vi "PH_ImageOperator.Show Beam Analysis.vi"(0 "i ref in":refnum<vi>, 2 "GUI Image In":T1, 5 "error in (no error)":errorcluster) -> (14 "i ref out":refnum<vi>, 16 "GUI Image Out":T1, 19 "error out":errorcluster)   [LabVIEW 2014, in "PH_ImageOperator.lvlib"]
doc: "This VI overlays beam analysis information to the GUI image."
uses:
  PH_ImageOperator.lvlib
  <vilib>/vision/Image Controls.llb/IMAQ Image.ctl
  PH_Image_Common/PH_Image_Common.lvlib
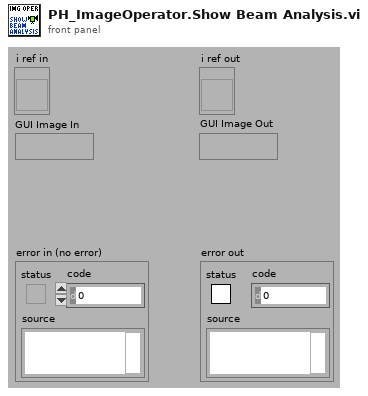
[diagram p1: front panel]
types:
  T1 = typedef "IMAQ Image.ctl" = refnum<image>
  T2 = typedef "PH_ImageOperator.lvlib/PH_ImageOperator.i attribute.ctl" = cluster{"GUI Refs":cluster{"Delete":refnum<vi>, "Calibration status":refnum<vi>, "BI subtracted":refnum<vi>, "calc Energy":refnum<vi>, "Energy: expected value":refnum<vi>, "Energy: Tolerance":refnum<vi>, "Energy calculated":refnum<vi>, "Energy":refnum<vi>, "calc Beam Anal":refnum<vi>, "Maj Diam 1/esquare":refnum<vi>, "Min Diam 1/esquare":refnum<vi>, "Azi Angle":refnum<vi>, "Min/Maj Diam esquare":refnum<vi>, "Beam analysed":refnum<vi>, "CoG - x":refnum<vi>, "CoG - y":refnum<vi>, "BA: Method":refnum<vi>, "BA: Steps":refnum<vi>, "BA: Factor":refnum<vi>, "calc Traces":refnum<vi>, "Traces: Fit Gauss":refnum<vi>, "Traces calculated":refnum<vi>, "Maj FWHM":refnum<vi>, "Min FWHM":refnum<vi>, "Major Trace":refnum<vi>, "Minor Trace":refnum<vi>, "Maj Fit Order":refnum<vi>, "Min Fit Order":refnum<vi>, "Position calculated":refnum<vi>, "Position":refnum<vi>, "Type":refnum<vi>, "Center":refnum<vi>, "exp - X":refnum<vi>, "exp - Y":refnum<vi>, "Tolerance":refnum<vi>, "f":refnum<vi>, "M":refnum<vi>, "D":refnum<vi>, "q":refnum<vi>, "Dummy Method":refnum<vi>, "Dummy Type":refnum<vi>, "Global On":refnum<vi>, "Traces: No offset":refnum<vi>, "Maj 99%":refnum<vi>, "Min 99%":refnum<vi>, "GUI FF Image":refnum<vi>, "calc Fill Factor":refnum<vi>, "FF calculated":refnum<vi>, "Fill Factor: Filter?":refnum<vi>, "FF: Damage Threshold":refnum<vi>, "FF: Threshold":refnum<vi>, "FF: max allow. Energy":refnum<vi>, "FF: Fillfactor":refnum<vi>, "Calibration data":refnum<vi>}, "List of GUIs":string[], "Calibration":cluster{"Status":T3, "Calibration data":T4, "Calibration Data File":path}, "Final Image":cluster{"BI Subtraction Failure":bool}, "Energy":cluster{"on":bool, "expected value [mJ]":dbl, "Tolerance [%]":dbl, "State":T3, "Energy [mJ]":dbl, "Unit":string, "calculated @":timestamp}, "Beam Analysis":cluster{"on":bool, "Data":T5, "Method":bool, "Steps":i32, "Factor":i32, "ROI":cluster{"Left":i32, "Top":i32, "Right":i32, "Bottom":i32}, "analysed @":timestamp}, "Trace Analysis":cluster{"on":bool, "Fit on":bool, "Maj FWHM":dbl, "Min FWHM":dbl, "Maj Fit Order":i32, "Min Fit Order":i32, "No Offset":bool, "Maj 99%":dbl, "Min 99%":dbl, "Traces":cluster{"XScaleName":string, "Y Scale Minimum":sgl, "Y Scale Maximum":sgl, "X Scale Minimum":sgl, "X Scale Maximum":sgl, "Traces":cluster{"Index":sgl[], "Trace":dbl[]}[]}[], "analysed @":timestamp}, "Position Analysis":cluster{"on":bool, "exp - X":i32, "exp - Y":i32, "focal length [mm]":dbl, "Magnification":dbl, "Delta":dbl, "Theta":dbl, "Tolerance":dbl, "Type":bool, "analysed @":timestamp}, "Fill Factor":cluster{"on":bool, "Filter on?":bool, "Threshold":dbl, "Damage Threshold [J/cm²]":dbl, "Fillfactor":dbl, "Max. allowed Energy [J]":dbl, "calculated @":timestamp}, "Statistician Service ID":i32, "Images":cluster{"Background":T1, "OP":T1, "GUI":T1, "BA: ROI":T1, "Trace: Turn":T1, "FF: Main":T1, "FF: Help":T1, "PSDB: BG":T1, "PSDB: OP":T1, "PSDB: FF":T1}}
  T3 = typedef "PH_StatusHandler.lvlib/PH_StatusHandler.Status.ctl" = i16
  T4 = typedef "PH_ImageCalibrator.lvlib/PH_ImageCalibrator.Calibration Data.ctl" = cluster{"Date":string, "Time":string, "Cam Settings":cluster{"Cam ID":string, "Gain":dbl, "Brightness":dbl, "Shutter":dbl, "Cam Error":bool, "Mode":i32}, "Background Image":cluster{"Image":dbl[][], "Image Error":bool}, "Linear Calibration":cluster{"Calibration Factor":dbl, "not mm or mrad":bool}, "Energy Calibration":cluster{"Calibration Factor":dbl, "no mJ":bool}}
  T5 = typedef "PH_ImageOperator.lvlib/PH_ImageOperator.Beam Analysis Data.ctl" = cluster{"CoG-x":sgl, "CoG-y":sgl, "Maj Dim":dbl, "Min Dim":dbl, "Ellipticity":dbl, "Azimuth Angle [rad]":dbl, "Azi Angle rel to Maj?":bool}
  T6 = cluster{"Left":i32, "Top":i32, "Right":i32, "Bottom":i32}
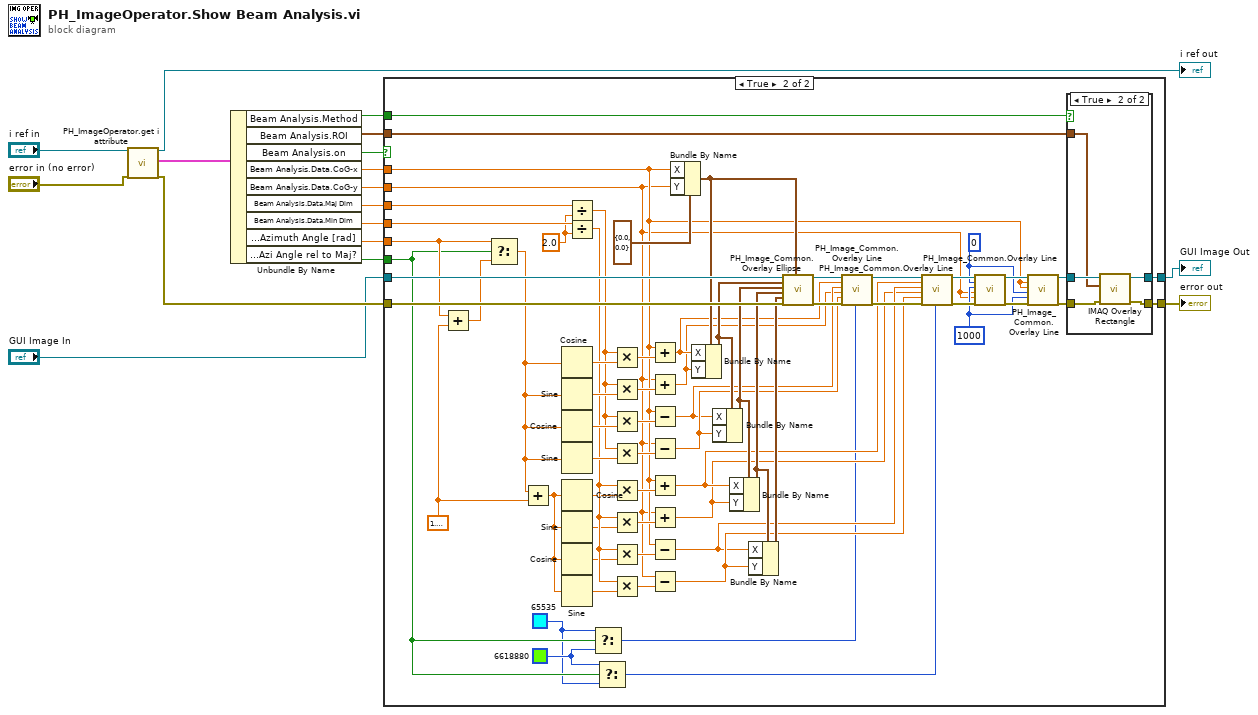
[diagram p0: block diagram]
diagram:
  n1 = call "PH_ImageOperator.get i attribute.vi"("i ref in"="i ref in", "error in (no error)"="error in (no error)") -> ("i ref out"=→"i ref out":refnum<vi>, "i attribute"=w3:T2, "error out"=w10:errorcluster)  [unwired: 15 in]
  n2 = Unbundle By Name(w3) -> ("Beam Analysis.Method"=w2:bool, "Beam Analysis.ROI"=w1:T6, "Beam Analysis.on"=w6:bool, "Beam Analysis.Data.CoG-x"=w14:sgl, "Beam Analysis.Data.CoG-y"=w13:sgl, "Beam Analysis.Data.Maj Dim"=w7:dbl, "Beam Analysis.Data.Min Dim"=w8:dbl, "Beam Analysis.Data.Azimuth Angle [rad]"=w5:dbl, "Beam Analysis.Data.Azi Angle rel to Maj?"=w4:bool)
  n3 = case shown="True" w6 {
    tunnel: w14 -> [_ w43]
    tunnel: w13 -> [_ w41]
    tunnel: [w18 w27] -> w12
    tunnel: [w19 w29] -> w11
    tunnel: w10 -> [w19 w83]
    tunnel: "GUI Image In" -> [w18 w84]
    tunnel: w8 -> [_ w49]
    tunnel: w7 -> [_ w51]
    tunnel: w5 -> [_ w38]
    tunnel: w4 -> [_ w23]
    tunnel: w2 -> [_ w26]
    tunnel: w1 -> [_ w25]
    frame False {
    }
    frame True {
      w37 = 1.5707963267948966
      w47 = sgl 2.0 ("y")
      w22 = u32 6618880 ("Color (red)")
      w21 = u32 65535 ("Color (red)")
      w52 = 1000 ("End x")
      w53 = 0 ("Start x")
      n4 = Add(x=w38, y=w37) -> (x+y=w36:dbl)
      n5 = Select(t=w38, s=w23, f=w36) -> (s? t:f=w39:dbl)
      n6 = Add(x=w39, y=w37) -> (x+y=w34:dbl)
      n7 = Cosine(x=w39) -> (cos(x)=w81:dbl)
      n8 = Sine(x=w39) -> (sin(x)=w79:dbl)
      n9 = Cosine(x=w39) -> (cos(x)=w75:dbl)
      n10 = Sine(x=w39) -> (sin(x)=w73:dbl)
      n11 = Cosine(x=w34) -> (cos(x)=w35:dbl)
      n12 = Sine(x=w34) -> (sin(x)=w33:dbl)
      n13 = Cosine(x=w34) -> (cos(x)=w32:dbl)
      n14 = Sine(x=w34) -> (sin(x)=w31:dbl)
      n15 = Divide(x=w51, y=w47) -> (x/y=w50:dbl)
      n16 = Divide(x=w49, y=w47) -> (x/y=w48:dbl)
      n17 = Select(t=w21, s=w23, f=w22) -> (s? t:f=w24:u32)
      n18 = Select(t=w22, s=w23, f=w21) -> (s? t:f=w20:u32)
      n19 = Multiply(x=w50, y=w81) -> (x*y=w82:dbl)
      n20 = Multiply(x=w50, y=w79) -> (x*y=w80:dbl)
      n21 = Multiply(x=w50, y=w75) -> (x*y=w76:dbl)
      n22 = Multiply(x=w50, y=w73) -> (x*y=w74:dbl)
      n23 = Multiply(x=w48, y=w35) -> (x*y=w72:dbl)
      n24 = Multiply(x=w48, y=w33) -> (x*y=w71:dbl)
      n25 = Multiply(x=w48, y=w32) -> (x*y=w70:dbl)
      n26 = Multiply(x=w48, y=w31) -> (x*y=w69:dbl)
      n27 = Add(x=w43, y=w82) -> (x+y=w42:dbl)
      n28 = Add(x=w41, y=w80) -> (x+y=w40:dbl)
      n29 = Subtract(x=w43, y=w76) -> (x-y=w46:dbl)
      n30 = Subtract(x=w41, y=w74) -> (x-y=w60:dbl)
      n31 = Add(x=w43, y=w72) -> (x+y=w59:dbl)
      n32 = Add(x=w41, y=w71) -> (x+y=w44:dbl)
      n33 = Subtract(x=w43, y=w70) -> (x-y=w45:dbl)
      n34 = Subtract(x=w41, y=w69) -> (x-y=w58:dbl)
      n35 = Bundle By Name(cluster=cluster{"X":sgl, "Y":sgl} {"X"=0.0, "Y"=0.0} ("COG Ellipse"), "X"=w43, "Y"=w41) -> (w68:cluster{"X":sgl, "Y":sgl})
      n36 = Bundle By Name(cluster=w68, "X"=w42, "Y"=w40) -> (w67:cluster{"X":sgl, "Y":sgl})
      n37 = Bundle By Name(cluster=w67, "X"=w46, "Y"=w60) -> (w66:cluster{"X":sgl, "Y":sgl})
      n38 = Bundle By Name(cluster=w66, "X"=w59, "Y"=w44) -> (w65:cluster{"X":sgl, "Y":sgl})
      n39 = Bundle By Name(cluster=w65, "X"=w45, "Y"=w58) -> (w77:cluster{"X":sgl, "Y":sgl})
      n40 = call "PH_Image_Common.Overlay Ellipse.vi"("Image"=w84, "Start Major Axis"=w67, "End Major Axis"=w66, "Start Minor Axis"=w65, "End Minor Axis"=w77, "error in (no error)"=w83, "COG Ellipse"=w68) -> ("Image Out"=w64:T1, "error out"=w63:errorcluster)  [unwired: 11 in]
      n41 = call "PH_Image_Common.Overlay Line.vi"("Image"=w64, "Start x"=w42, "End x"=w46, "Start y"=w40, "End y"=w60, "error in (no error)"=w63, "Color (red)"=w24) -> ("Image Out"=w62:T1, "error out"=w61:errorcluster)  [unwired: 11 in]
      n42 = call "PH_Image_Common.Overlay Line.vi"("Image"=w62, "Start x"=w59, "End x"=w45, "Start y"=w44, "End y"=w58, "error in (no error)"=w61, "Color (red)"=w20) -> ("Image Out"=w57:T1, "error out"=w56:errorcluster)  [unwired: 11 in]
      n43 = call "PH_Image_Common.Overlay Line.vi"("Image"=w57, "Start x"=w53, "End x"=w52, "Start y"=w41, "End y"=w41, "error in (no error)"=w56) -> ("Image Out"=w55:T1, "error out"=w54:errorcluster)  [unwired: 12 in]
      n44 = call "PH_Image_Common.Overlay Line.vi"("Image"=w55, "Start x"=w43, "End x"=w43, "Start y"=w53, "End y"=w52, "error in (no error)"=w54) -> ("Image Out"=w28:T1, "error out"=w30:errorcluster)  [unwired: 12 in]
      n45 = case shown="True" w26 {
        tunnel: w30 -> [w85 w91]
        tunnel: [w85 w90] -> w29
        tunnel: w28 -> [w86 w89]
        tunnel: [w86 w88] -> w27
        tunnel: w25 -> [_ w87]
        frame False {
        }
        frame True {
          n46 = call "IMAQ Overlay Rectangle"("error in (no error)"=w91, "Rectangle"=w87, "Image"=w89) -> ("error out"=w90:errorcluster, "Image Out"=w88:T1)  [unwired: 7 in]
        }
      }
    }
  }
  "error out" <- w11
  "GUI Image Out" <- w12
